vi "215.InitializeSyringe (SubVI).vi"(8 "error in (no error)":errorcluster, 11 "VISA resource name":refnum<visa-resource-name>="COM7") -> (0 "error out":errorcluster, 1 "Receive string":string, 2 "Connected":bool, 3 "VISA Out":refnum<visa-resource-name>)   [LabVIEW 2017]
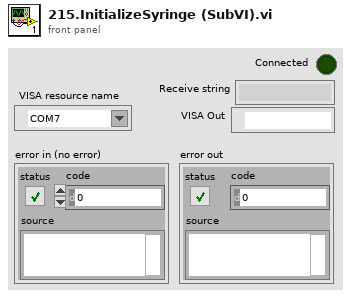
[diagram p1: front panel]
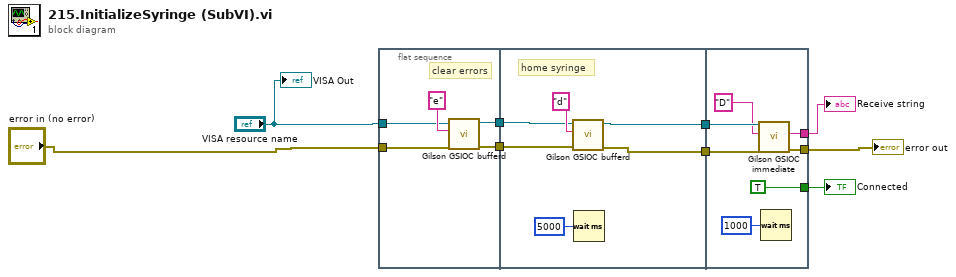
[diagram p0: block diagram]
diagram:
  n1 = flat-sequence {
    tunnel: "error in (no error)" -> [w13]
    tunnel: "VISA resource name" -> [w11]
    tunnel: [w12] -> w8
    tunnel: [w10] -> w9
    tunnel: [w20] -> w7
    tunnel: [w19] -> w6
    tunnel: w9 -> [w16]
    tunnel: w8 -> [w17]
    tunnel: [TRUE] -> w5
    tunnel: w7 -> [w26]
    tunnel: w6 -> [w25]
    tunnel: [w23] -> w1
    tunnel: [w21] -> w4
    frame #0 {
      # "clear errors"
      n2 = call <instrlib>:"Gilson GSIOC bufferd.vi"("error in (no error)"=w13, "Bufferd command"="e", "VISA resource name"=w11) -> ("error out"=w12:errorcluster, "VISA resource name out"=w10:refnum<visa-resource-name>)  [unwired: 6 in, 1 out]
    }
    frame #1 {
      # "home syringe"
      n3 = call <instrlib>:"Gilson GSIOC bufferd.vi"("error in (no error)"=w17, "Bufferd command"="d", "VISA resource name"=w16) -> ("error out"=w19:errorcluster, "VISA resource name out"=w20:refnum<visa-resource-name>)  [unwired: 6 in, 1 out]
      n4 = Wait (ms)(milliseconds to wait=u32 5000) -> ()  [unwired: 1 out]
    }
    frame #2 {
      n5 = call <instrlib>:"Gilson GSIOC immediate.vi"("error in (no error)"=w25, "Immediate command"="D", "VISA resource name"=w26) -> ("error out"=w23:errorcluster, "Receive string"=w21:string)  [unwired: 6 in, 1 out]
      n6 = Wait (ms)(milliseconds to wait=u32 1000) -> ()  [unwired: 1 out]
    }
  }
  "error out" <- w1
  "Connected" <- w5
  "VISA Out" <- "VISA resource name"
  "Receive string" <- w4
